vi "IOScan_InitScrollBar.vi"(8 "error in":errorcluster, 9 "Further Config Data":T1[](array[typedef]) {"Fault Config Choice" items=["Ignore", "Minor", "Major", "Custom", "Unconfigured"]; "Level After Threshold" items=["Ignore", "Minor", "Major"]; "Level Before Threshold" items=["Ignore", "Minor", "Major"]}, 10 "Configurable Faults in":refnum<vi>, 11 "Configurable Faults Scrollbar in":refnum<vi>) -> (0 "error out":errorcluster, 2 "Configurable Faults out":refnum<vi>, 3 "Configurable Faults Scrollbar out":refnum<vi>)   [LabVIEW 2016]
uses:
  <resource>/dialog/TargetPreferencePages/IOScan_SubVIs/IOScan_ConfigDataEntry.ctl
  <resource>/dialog/TargetPreferencePages/IOScan_SubVIs/IOScan_FaultLevel.ctl
  <resource>/dialog/TargetPreferencePages/IOScan_SubVIs/IOScan_FaultConfigChoice.ctl
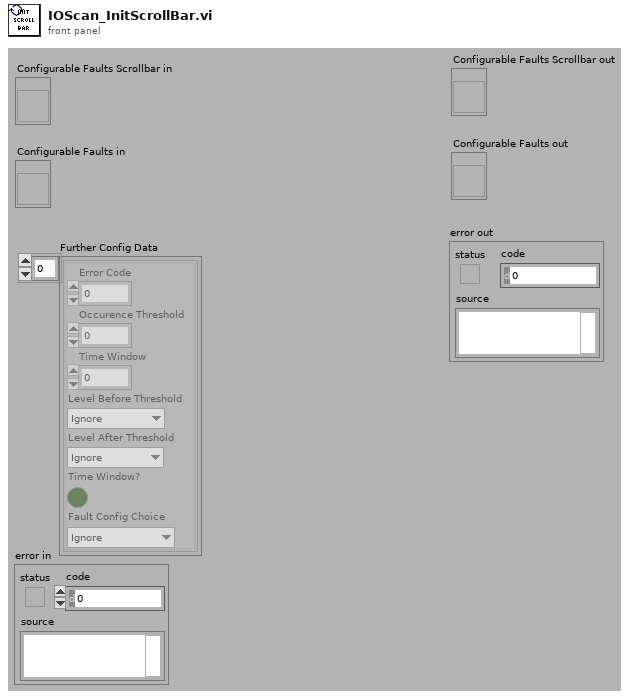
[diagram p1: front panel]
types:
  T1 = typedef "IOScan_ConfigDataEntry.ctl" = cluster{"Error Code":i32, "Occurence Threshold":u32, "Time Window":i32, "Level Before Threshold":T2, "Level After Threshold":T2, "Time Window?":bool, "Fault Config Choice":T3}
  T2 = typedef "IOScan_FaultLevel.ctl" = i32
  T3 = typedef "IOScan_FaultConfigChoice.ctl" = u16
  T4 = typedef "LVRectTypeDef.ctl" = cluster{"Left":i16, "Top":i16, "Right":i16, "Bottom":i16}
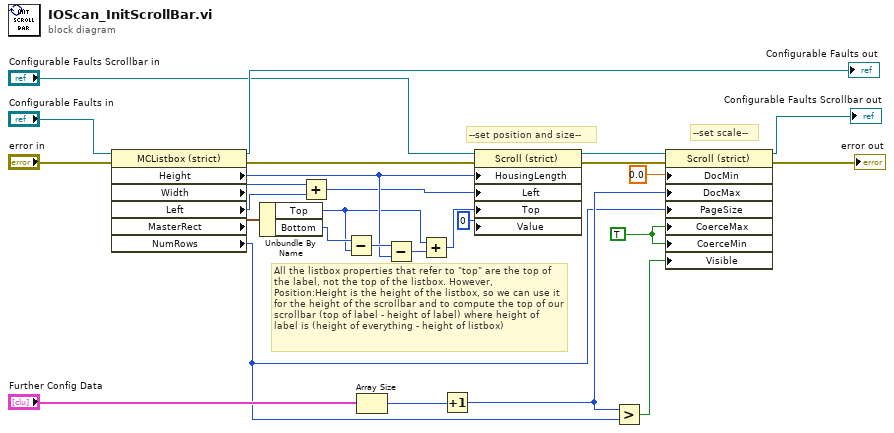
[diagram p0: block diagram]
diagram:
  w17 = TRUE ("Coerce Maximum Value")
  # "--set scale--"
  # "--set position and size--"
  # "All the listbox properties that refer to \"top\" are the top of the label, not the top of the listbox. However, Position:Height is the height of the listbox, so we can use it for the height of the scrollbar and to compute the top of our scrollbar (top of label - height of label) where height of label is (height of everything - height of listbox)"
  n1 = property class="MCListbox (strict)"(reference="Configurable Faults in", error in="error in") -> (reference out=→"Configurable Faults out":refnum<vi>, error out=w10:errorcluster, "Height"=w6:u32, "Width"=w11:u32, "Left"=w12:i32, "MasterRect"=w9:T4, "NumRows"=w2:u32)
  n2 = Unbundle By Name(w9) -> ("Top"=w4:i16, "Bottom"=w8:i16)
  n3 = Add(x=w11, y=w12) -> (x+y=w1:u32)
  n4 = Subtract(x=w8, y=w4) -> (x-y=w7:i16)
  n5 = Array Size(array="Further Config Data") -> (size(s)=w14:i32)
  n6 = Subtract(x=w7, y=w6) -> (x-y=w5:u32)
  n7 = Add(x=w4, y=w5) -> (x+y=w3:u32)
  n8 = Increment(x=w14) -> (x+1=w15:i32)
  n9 = property class="Scroll (strict)"(reference="Configurable Faults Scrollbar in", error in=w10, "HousingLength"=w6, "Left"=w1, "Top"=w3, "Value"=0) -> (reference out=w18:refnum<vi>, error out=w19:errorcluster)
  n10 = Greater?(x=w15, y=w2) -> (0:w16:bool)
  n11 = property class="Scroll (strict)"(reference=w18, error in=w19, "DocMin"=0.0 ("Doc Min"), "DocMax"=w15, "PageSize"=w2, "CoerceMax"=w17, "CoerceMin"=w17, "Visible"=w16) -> (reference out=→"Configurable Faults Scrollbar out":refnum<vi>, error out=→"error out":errorcluster)
